vi "实验5 相移键控RX.vi"() -> ()   [LabVIEW 2015]
uses:
  SubVI/SubVI RX HW Parameters.ctl
  SubVI/SubVI TX Synchronization Params.ctl
  <vilib>/addons/Modulation/Analog/controls/Complex Data Waveform.ctl
  <vilib>/addons/Modulation/Analog/support/Validators/mod_Fractional Resample Validate.vi
  <vilib>/addons/Modulation/Analog/support/Validators/mod_Check Flush State.vi
  <vilib>/addons/Modulation/Analog/support/mod_FractionalResampler.vi
  <vilib>/addons/Modulation/Analog/support/mod_Integer Rate Interpolation.vi
  <vilib>/addons/Modulation/Analog/support/mod_Set Error Source.vi
  <vilib>/addons/Modulation/Analog/support/Validators/mod_Validate Complex Waveform.vi
  <vilib>/addons/Modulation/Analog/support/mod_PerformResampling.vi
  <vilib>/addons/Modulation/Analog/support/Validators/mod_WFErrorHandler.vi
  <vilib>/Utility/error.llb/Error Cluster From Error Code.vi
  <vilib>/addons/Modulation/Analog/support/mod_Resampling Factors.vi
  <vilib>/addons/Modulation/Analog/support/mod_ResamplingFilter.vi
  <vilib>/addons/Modulation/Analog/support/mod_Generate Integer Interpolation Filter.vi
  <vilib>/addons/Modulation/niAMT.lvlib
panel:
  out "接收文本":string
  out "误码率曲线":dbl(graph)
  in  "图形选项卡":enum32{"信号星座图", "信号眼图", "信号IQ波形"}(tab)=enum."信号IQ波形"
  out "信号星座图":cluster{dbl[], dbl[]}(graph)
  out "信号眼图":cluster{"t0":dbl, "dt":dbl, "Y":dbl[]}[](graph)
  out "输出I波形":waveform(dbl)(graph)
  out "输出Q波形":waveform(dbl)(graph)
  out "接收状态":bool=TRUE
  in  "停止":bool
  out "当前状态":string="接收机关闭"
  in  "设置选项卡":enum32{"硬件设置", "调制设置", "同步设置 ", "调试"}(tab)
  in  "硬件设置":T1={"设备IP地址"="192.168.10.2", "选择天线"="RX2", "载波频率(Hz)"=800000000.0, "增益(dB)"=10.0, "采样时间(s)"=0.035, "触发电平"=0.01, "带宽(Hz)"=40000000.0, "参考位置(%)"=10.0} {"参考位置(%)" format="%.2p"; "带宽(Hz)" format="%.2p"; "触发电平" format="%.2p"; "采样时间(s)" format="%.2p"; "增益(dB)" format="%.2f"; "载波频率(Hz)" format="%.2p"}
  in  "调制设置":T2={"调制方式"="QPSK", "脉冲成型参数"={"调制方式"=enum."PSK", "脉冲成型滤波器"=enum."根升余弦", "滤波器参数"=0.5, "滤波长度 (码元)"=8}, "RX  过采样因子"=4, "RX 采样率"=500000.0} {"RX 采样率" items=["25M"=25000000.0, "20M"=20000000.0, "16.6667M"=16666666.666667, "14.2857M"=14285714.285714, "12.5M"=12500000.0, "11.1111M"=11111111.111111, "10M"=10000000.0, "9.09091M"=9090909.090909, "8.33333M"=8333333.333333, "7.69231M"=7692307.692308, "7.14286M"=7142857.142857, "6.66667M"=6666666.666667, "6.25M"=6250000.0, "5.88235M"=5882352.941176, "5.55556M"=5555555.555556, "5.26316M"=5263157.894737, "5M"=5000000.0, "4.7619M"=4761904.761905, "4.54545M"=4545454.545455, "4.34783M"=4347826.086957, "4.16667M"=4166666.666667, "4M"=4000000.0, "3.84615M"=3846153.846154, "3.7037M"=3703703.703704, "3.57143M"=3571428.571429, "3.44828M"=3448275.862069, "3.33333M"=3333333.333333, "3.22581M"=3225806.451613, "3.125M"=3125000.0, "3.0303M"=3030303.030303, "2.94118M"=2941176.470588, "2.85714M"=2857142.857143, "2.77778M"=2777777.777778, "2.7027M"=2702702.702703, "2.63158M"=2631578.947368, "2.5641M"=2564102.564103, "2.5M"=2500000.0, "2.43902M"=2439024.390244, "2.38095M"=2380952.380952, "2.32558M"=2325581.395349, "2.27273M"=2272727.272727, "2.22222M"=2222222.222222, "2.17391M"=2173913.043478, "2.12766M"=2127659.574468, "2.08333M"=2083333.333333, "2.04082M"=2040816.326531, "2M"=2000000.0, "1.96078M"=1960784.313725, "1.92308M"=1923076.923077, "1.88679M"=1886792.45283, "1.85185M"=1851851.851852, "1.81818M"=1818181.818182, "1.78571M"=1785714.285714, "1.75439M"=1754385.964912, "1.72414M"=1724137.931034, "1.69492M"=1694915.254237, "1.66667M"=1666666.666667, "1.63934M"=1639344.262295, "1.6129M"=1612903.225806, "1.5873M"=1587301.587302, "1.5625M"=1562500.0, "1.53846M"=1538461.538462, "1.51515M"=1515151.515152, "1.49254M"=1492537.313433, "1.47059M"=1470588.235294, "1.44928M"=1449275.362319, "1.42857M"=1428571.428571, "1.40845M"=1408450.704225, "1.38889M"=1388888.888889, "1.36986M"=1369863.013699, "1.35135M"=1351351.351351, "1.33333M"=1333333.333333, "1.31579M"=1315789.473684, "1.2987M"=1298701.298701, "1.28205M"=1282051.282051, "1.26582M"=1265822.78481, "1.25M"=1250000.0, "1.23457M"=1234567.901235, "1.21951M"=1219512.195122, "1.20482M"=1204819.277108, "1.19048M"=1190476.190476, "1.17647M"=1176470.588235, "1.16279M"=1162790.697674, "1.14943M"=1149425.287356, "1.13636M"=1136363.636364, "1.1236M"=1123595.505618, "1.11111M"=1111111.111111, "1.0989M"=1098901.098901, "1.08696M"=1086956.521739, "1.07527M"=1075268.817204, "1.06383M"=1063829.787234, "1.05263M"=1052631.578947, "1.04167M"=1041666.666667, "1.03093M"=1030927.835052, "1.02041M"=1020408.163265, "1.0101M"=1010101.010101, "1M"=1000000.0, "990.099k"=990099.009901, "980.392k"=980392.156863, "970.874k"=970873.786408, "961.538k"=961538.461538, "952.381k"=952380.952381, "943.396k"=943396.226415, "934.579k"=934579.439252, "925.926k"=925925.925926, "917.431k"=917431.192661, "909.091k"=909090.909091, "900.901k"=900900.900901, "892.857k"=892857.142857, "884.956k"=884955.752212, "877.193k"=877192.982456, "869.565k"=869565.217391, "862.069k"=862068.965517, "854.701k"=854700.854701, "847.458k"=847457.627119, "840.336k"=840336.134454, "833.333k"=833333.333333, "826.446k"=826446.280992, "819.672k"=819672.131148, "813.008k"=813008.130081, "806.452k"=806451.612903, "800k"=800000.0, "793.651k"=793650.793651, "787.402k"=787401.574803, "781.25k"=781250.0, "769.231k"=769230.769231, "757.576k"=757575.757576, "746.269k"=746268.656716, "735.294k"=735294.117647, "724.638k"=724637.681159, "714.286k"=714285.714286, "704.225k"=704225.352113, "694.444k"=694444.444444, "684.932k"=684931.506849, "675.676k"=675675.675676, "666.667k"=666666.666667, "657.895k"=657894.736842, "649.351k"=649350.649351, "641.026k"=641025.641026, "632.911k"=632911.392405, "625k"=625000.0, "617.284k"=617283.950617, "609.756k"=609756.097561, "602.41k"=602409.638554, "595.238k"=595238.095238, "588.235k"=588235.294118, "581.395k"=581395.348837, "574.713k"=574712.643678, "568.182k"=568181.818182, "561.798k"=561797.752809, "555.556k"=555555.555556, "549.451k"=549450.549451, "543.478k"=543478.26087, "537.634k"=537634.408602, "531.915k"=531914.893617, "526.316k"=526315.789474, "520.833k"=520833.333333, "515.464k"=515463.917526, "510.204k"=510204.081633, "505.051k"=505050.505051, "500k"=500000.0, "495.05k"=495049.50495, "490.196k"=490196.078431, "485.437k"=485436.893204, "480.769k"=480769.230769, "476.19k"=476190.47619, "471.698k"=471698.113208, "467.29k"=467289.719626, "462.963k"=462962.962963, "458.716k"=458715.59633, "454.545k"=454545.454545, "450.45k"=450450.45045, "446.429k"=446428.571429, "442.478k"=442477.876106, "438.596k"=438596.491228, "434.783k"=434782.608696, "431.034k"=431034.482759, "427.35k"=427350.42735, "423.729k"=423728.813559, "420.168k"=420168.067227, "416.667k"=416666.666667, "413.223k"=413223.140496, "409.836k"=409836.065574, "406.504k"=406504.065041, "403.226k"=403225.806452, "400k"=400000.0, "396.825k"=396825.396825, "393.701k"=393700.787402, "390.625k"=390625.0, "384.615k"=384615.384615, "378.788k"=378787.878788, "373.134k"=373134.328358, "367.647k"=367647.058824, "362.319k"=362318.84058, "357.143k"=357142.857143, "352.113k"=352112.676056, "347.222k"=347222.222222, "342.466k"=342465.753425, "337.838k"=337837.837838, "333.333k"=333333.333333, "328.947k"=328947.368421, "324.675k"=324675.324675, "320.513k"=320512.820513, "316.456k"=316455.696203, "312.5k"=312500.0, "308.642k"=308641.975309, "304.878k"=304878.04878, "301.205k"=301204.819277, "297.619k"=297619.047619, "294.118k"=294117.647059, "290.698k"=290697.674419, "287.356k"=287356.321839, "284.091k"=284090.909091, "280.899k"=280898.876404, "277.778k"=277777.777778, "274.725k"=274725.274725, "271.739k"=271739.130435, "268.817k"=268817.204301, "265.957k"=265957.446809, "263.158k"=263157.894737, "260.417k"=260416.666667, "257.732k"=257731.958763, "255.102k"=255102.040816, "252.525k"=252525.252525, "250k"=250000.0, "247.525k"=247524.752475, "245.098k"=245098.039216, "242.718k"=242718.446602, "240.385k"=240384.615385, "238.095k"=238095.238095, "235.849k"=235849.056604, "233.645k"=233644.859813, "231.481k"=231481.481481, "229.358k"=229357.798165, "227.273k"=227272.727273, "225.225k"=225225.225225, "223.214k"=223214.285714, "221.239k"=221238.938053, "219.298k"=219298.245614, "217.391k"=217391.304348, "215.517k"=215517.241379, "213.675k"=213675.213675, "211.864k"=211864.40678, "210.084k"=210084.033613, "208.333k"=208333.333333, "206.612k"=206611.570248, "204.918k"=204918.032787, "203.252k"=203252.03252, "201.613k"=201612.903226, "200k"=200000.0, "198.413k"=198412.698413, "196.85k"=196850.393701, "195.312k"=195312.5]}
  in  "同步设置":T3={"码元数据量 (源)"=2660, "训练队列(源)"=[0.7071067811865475+0.7071067811865475i, 0.7071067811865475+0.7071067811865475i, 0.7071067811865475+0.7071067811865475i, -0.7071067811865475-0.7071067811865475i, -0.7071067811865475-0.7071067811865475i, -0.7071067811865475-0.7071067811865475i, 0.7071067811865475+0.7071067811865475i, -0.7071067811865475-0.7071067811865475i, -0.7071067811865475-0.7071067811865475i, 0.7071067811865475+0.7071067811865475i, -0.7071067811865475-0.7071067811865475i, 0.7071067811865475+0.7071067811865475i, 0.7071067811865475+0.7071067811865475i, 0.7071067811865475+0.7071067811865475i, -0.7071067811865475-0.7071067811865475i, -0.7071067811865475-0.7071067811865475i, -0.7071067811865475-0.7071067811865475i, 0.7071067811865475+0.7071067811865475i, -0.7071067811865475-0.7071067811865475i, -0.7071067811865475-0.7071067811865475i, 0.7071067811865475+0.7071067811865475i, -0.7071067811865475-0.7071067811865475i, 0.7071067811865475+0.7071067811865475i, 0.7071067811865475+0.7071067811865475i, 0.7071067811865475+0.7071067811865475i, -0.7071067811865475-0.7071067811865475i, -0.7071067811865475-0.7071067811865475i, -0.7071067811865475-0.7071067811865475i, 0.7071067811865475+0.7071067811865475i, -0.7071067811865475-0.7071067811865475i, -0.7071067811865475-0.7071067811865475i, 0.7071067811865475+0.7071067811865475i, -0.7071067811865475-0.7071067811865475i, 0.7071067811865475+0.7071067811865475i, 0.7071067811865475+0.7071067811865475i, 0.7071067811865475+0.7071067811865475i, -0.7071067811865475-0.7071067811865475i, -0.7071067811865475-0.7071067811865475i, -0.7071067811865475-0.7071067811865475i, 0.7071067811865475+0.7071067811865475i, -0.7071067811865475-0.7071067811865475i, -0.7071067811865475-0.7071067811865475i, 0.7071067811865475+0.7071067811865475i, -0.7071067811865475-0.7071067811865475i], "补零长度"=8, "同步方式"="Timing Estimation", "码元定时恢复算法"="Max Energy", "帧检测算法"="Self Reference w/Power Normalization", "修正频偏"=FALSE}
  out "强制载波频率(Hz)":dbl=800000000.0 format="%#_6p"
  out "强制IQ速率":dbl=500000.0 format="%#_6p"
  out "强制增益(dB)":dbl=10.0 format="%#_6f"
  out "强制带宽":dbl=32000000.0
  # "实验5 相移键控RX"
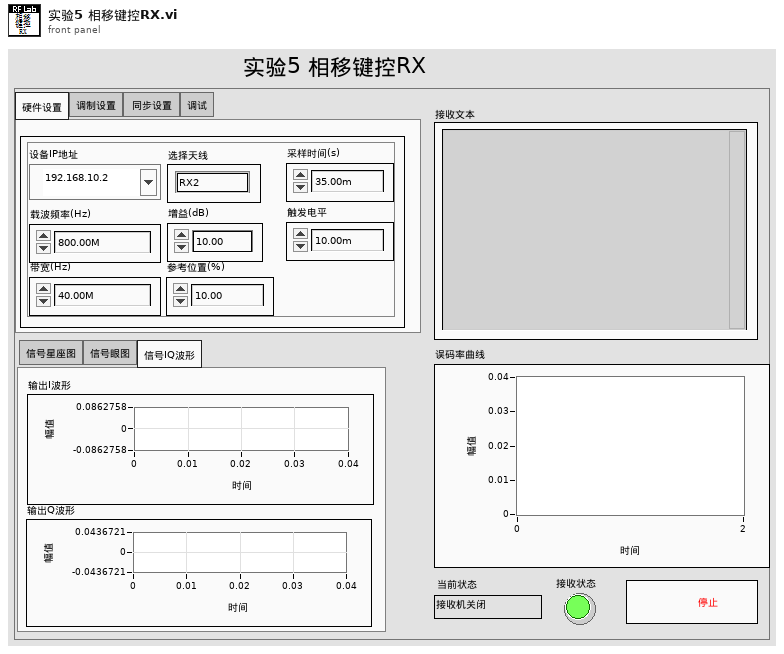
[diagram p1: front panel]
types:
  T1 = typedef "SubVI RX HW Parameters.ctl" = cluster{"设备IP地址":refnum<k15>, "选择天线":string, "载波频率(Hz)":dbl, "增益(dB)":dbl, "采样时间(s)":dbl, "触发电平":dbl, "带宽(Hz)":dbl, "参考位置(%)":dbl}
  T2 = cluster{"调制方式":string, "脉冲成型参数":cluster{"调制方式":enum16{"FSK", "PSK", "QAM", "MSK", "PAM", "ASK"}, "脉冲成型滤波器":enum16{"无", "升余弦", "根升余弦", "高斯"}, "滤波器参数":dbl, "滤波长度 (码元)":i32}, "RX  过采样因子":i32, "RX 采样率":dbl}
  T3 = typedef "SubVI TX Synchronization Params.ctl" = cluster{"码元数据量 (源)":i32, "训练队列(源)":cdb[], "补零长度":i32, "同步方式":string, "码元定时恢复算法":string, "帧检测算法":string, "修正频偏":bool}
  T4 = typedef "niAMT.lvlib/Complex Data Waveform.ctl" = cluster{"t0":dbl, "dt":dbl, "Y":cdb[]}
  T5 = typedef "SubVI RX Modulation Simple Params.ctl" = cluster{"调制方式":string, "脉冲成型参数":cluster{"调制方式":enum16{"FSK", "PSK", "QAM", "MSK", "PAM", "ASK"}, "脉冲成型滤波器":enum16{"无", "升余弦", "根升余弦", "高斯"}, "滤波器参数":dbl, "滤波长度 (码元)":i32}, "RX  过采样因子":i32, "RX 采样率":dbl}
  T6 = cluster{"Constellation Graph":cluster{dbl[], dbl[]}, "eye diagram":cluster{"t0":dbl, "dt":dbl, "Y":dbl[]}[], "Power Delay Profile":waveform(dbl)}
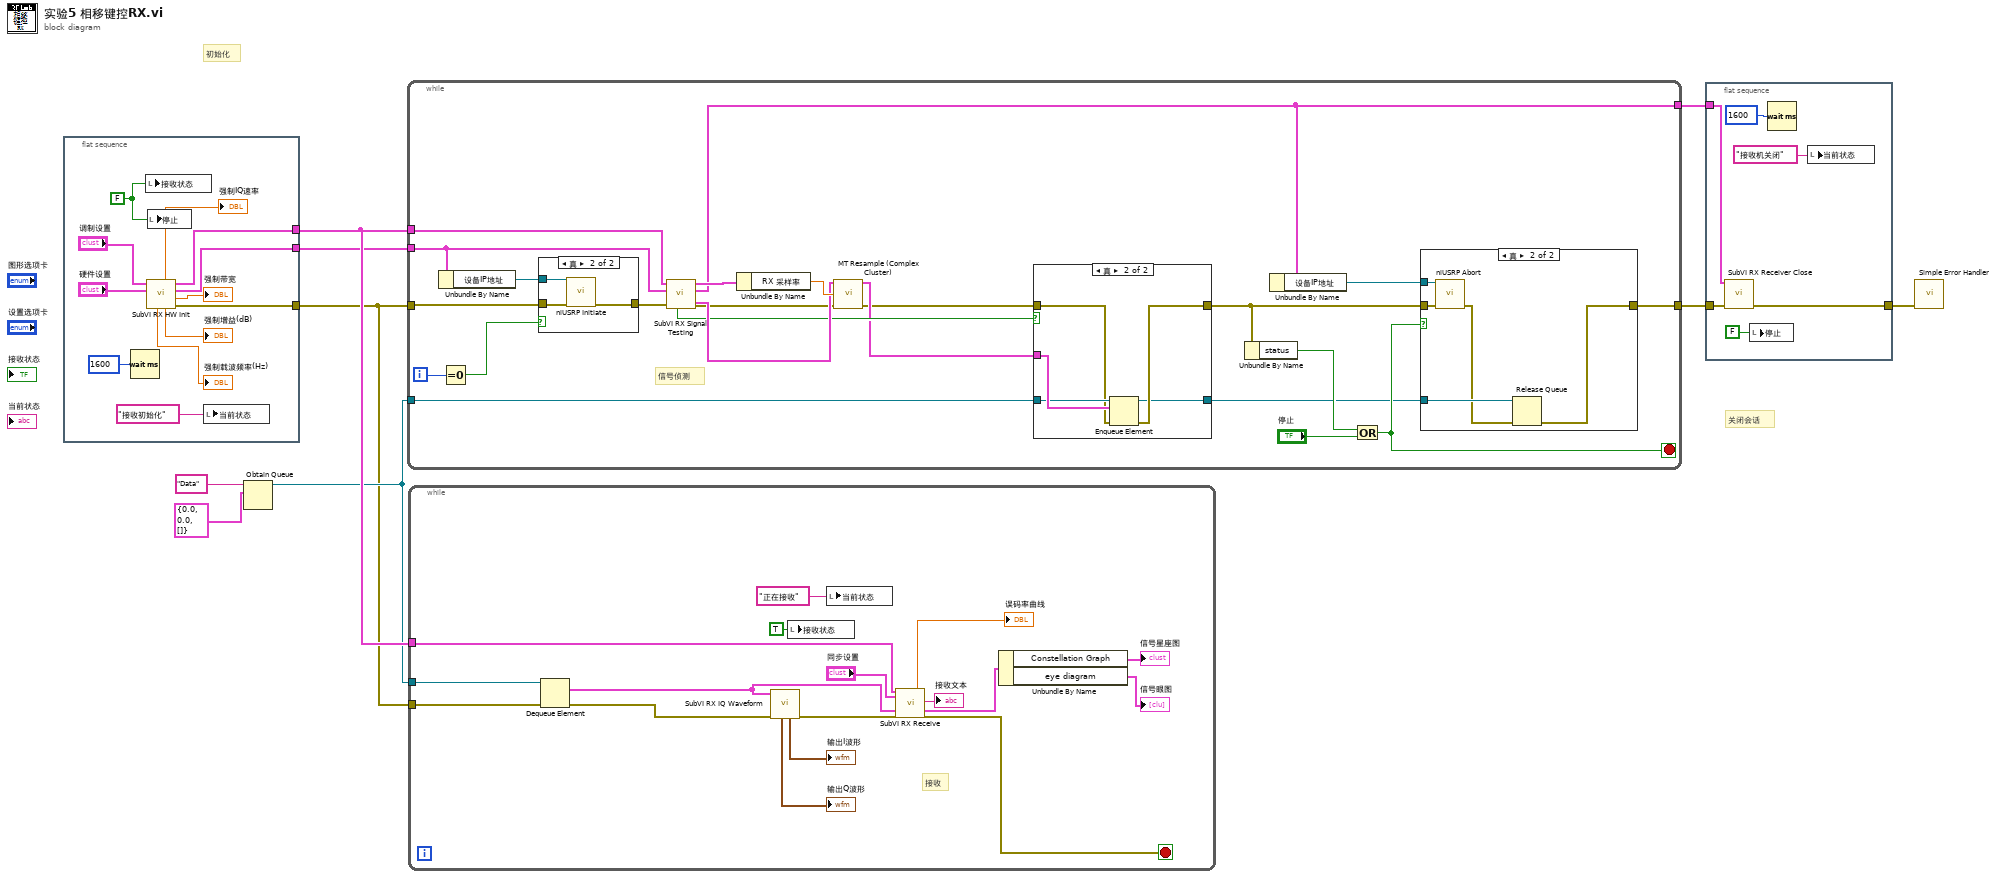
[diagram p0: block diagram]
diagram:
  # "关闭会话"
  # "初始化"
  n1 = flat-sequence {
    tunnel: [w14] -> w6
    tunnel: [w13] -> w5
    tunnel: [w12] -> w1
    frame #0 {
      w10 = FALSE ("接收？")
      n2 = Wait (ms)(milliseconds to wait=u32 1600 ("等待时间（毫秒）")) -> ()  [unwired: 1 out]
      n3 = local write "接收状态"(w10) -> ()
      n4 = call "SubVI RX HW Init.vi"("硬件设置"="硬件设置", "调制设置"="调制设置") -> ("错误输出"=w12:errorcluster, "强制带宽"=→"强制带宽":dbl, "硬件设置"=w13:T1, "调制设置"=w14:T5, "强制增益(dB)"=→"强制增益(dB)":dbl, "强制IQ速率"=→"强制IQ速率":dbl, "强制载波频率(Hz)"=→"强制载波频率(Hz)":dbl)  [unwired: 3 in]
      n5 = local write "停止"(w10) -> ()
      n6 = local write "当前状态"("接收初始化" ("当前状态")) -> ()
    }
  }
  n7 = Obtain Queue(name (unnamed)="Data" ("名称（未命名）"), element data type=T4 {"t0"=0.0, "dt"=0.0, "Y"=[]} ("output complex waveform")) -> (queue out=w2:refnum<queue>)  [unwired: 3 in, 2 out]
  n8 = while {
    tunnel: w6 -> [w34]
    tunnel: w5 -> [w33]
    tunnel: w1 -> [w38]
    tunnel: [w29] -> w9
    tunnel: [w31] -> w8
    tunnel: w2 -> [w25]
    i -> [w36]
    stop <- w30 stop-if-true
    # "信号侦测"
    n9 = Unbundle By Name(w33) -> ("设备IP地址"=w32:refnum<k15>)
    n10 = Equal To 0?(x=w36) -> (x = 0?=w35:bool)
    n11 = case shown="真" w35 {
      tunnel: w38 -> [w58 w61]
      tunnel: [w58 w60] -> w37
      tunnel: w32 -> [_ w59]
      frame False {
      }
      frame True {
        n12 = call <instrlib>:"niUSRP Initiate.vi"("session handle"=w59, "error in (no error)"=w61) -> ("error out"=w60:errorcluster)  [unwired: 12 in, 1 out]
      }
    }
    n13 = call "SubVI RX Signal Testing.vi"("错误输入"=w37, "硬件设置"=w33, "调制设置"=w34) -> ("错误输出"=w42:errorcluster, "硬件设置"=w29:T1, "调制设置"=w41:T5, "接收IQ波形"=w43:cluster{"t0":dbl, "dt":dbl, "Y":cdb[]}, "数据包检测"=w27:bool)  [unwired: 4 in]
    n14 = Unbundle By Name(w41) -> ("RX 采样率"=w44:dbl)
    n15 = call <vilib>:"MT Resample (Complex Cluster).vi"("input complex waveform"=w43, "desired sample rate (Hz)"=w44, "error in (no error)"=w42) -> ("output complex waveform"=w26:T4, "error out"=w24:errorcluster)  [unwired: 11 in]
    n16 = case shown="真" w27 {
      tunnel: w26 -> [_ w51]
      tunnel: w25 -> [w45 w50]
      tunnel: w24 -> [w46 w49]
      tunnel: [w46 w48] -> w23
      tunnel: [w45 w47] -> w22
      frame False {
      }
      frame True {
        n17 = Enqueue Element(queue=w50, element=w51, error in (no error)=w49) -> (queue out=w47:refnum<queue>, error out=w48:errorcluster)  [unwired: 1 in, 1 out]
      }
    }
    n18 = Unbundle By Name(w23) -> ("status"=w40:bool)
    n19 = Unbundle By Name(w29) -> ("设备IP地址"=w28:refnum<k15>)
    n20 = Or(x=w40, y="停止") -> (x .or. y?=w30:bool)
    n21 = case shown="真" w30 {
      tunnel: w23 -> [w52 w57]
      tunnel: [w52 w53] -> w31
      tunnel: w28 -> [_ w56]
      tunnel: w22 -> [_ w55]
      frame False {
      }
      frame True {
        n22 = call <instrlib>:"niUSRP Abort.vi"("session handle"=w56, "error in (no error)"=w57) -> ("error out"=w54:errorcluster)  [unwired: 12 in, 1 out]
        n23 = Release Queue(queue=w55, error in (no error)=w54) -> (error out=w53:errorcluster)  [unwired: 1 in, 2 out]
      }
    }
  }
  n24 = while {
    tunnel: w6 -> [w78]
    tunnel: w2 -> [w77]
    tunnel: w1 -> [w74]
    stop <- w62 stop-if-true
    # "接收"
    n25 = Dequeue Element(queue=w77, error in (no error)=w74) -> (element=w76:T4, error out=w75:errorcluster)  [unwired: 1 in, 2 out]
    n26 = call "SubVI RX IQ Waveform.vi"("错误输入"=w75, "接收IQ波形"=w76) -> ("错误输出"=w69:errorcluster, "I"=→"输出I波形":waveform(dbl), "Q"=→"输出Q波形":waveform(dbl))  [unwired: 7 in]
    n27 = local write "接收状态"(TRUE ("接收？")) -> ()
    n28 = local write "当前状态"("正在接收" ("当前状态")) -> ()
    n29 = call "SubVI RX Receive.vi"("调制设置"=w78, "同步设置"="同步设置", "输入复杂波形"=w76, "错误输入"=w69) -> ("误码率"=→"误码率曲线":dbl, "信息恢复"=→"接收文本":string, "RX波形输出"=w68:T6, "错误输出"=w62:errorcluster)  [unwired: 11 in, 1 out]
    n30 = Unbundle By Name(w68) -> ("Constellation Graph"=→"信号星座图":cluster{dbl[], dbl[]}, "eye diagram"=→"信号眼图":cluster{"t0":dbl, "dt":dbl, "Y":dbl[]}[])
  }
  n31 = flat-sequence {
    tunnel: w9 -> [w83]
    tunnel: w8 -> [w82]
    tunnel: [w81] -> w7
    frame #0 {
      n32 = call "SubVI RX Receiver Close.vi"("硬件设置"=w83, "错误输入"=w82) -> ("错误输出"=w81:errorcluster)  [unwired: 13 in]
      n33 = local write "停止"(FALSE ("接收？")) -> ()
      n34 = Wait (ms)(milliseconds to wait=u32 1600 ("等待时间（毫秒）")) -> ()  [unwired: 1 out]
      n35 = local write "当前状态"("接收机关闭" ("当前状态")) -> ()
    }
  }
  n36 = call <vilib>:"Simple Error Handler.vi"("error in (no error)"=w7) -> ()  [unwired: 4 in, 5 out]
